vi "GSP_Manager_SCLNServer_Handler.vi"(4 "error in (no error)":errorcluster, 6 "Actions":T1) -> (0 "error out":errorcluster, 2 "reference out (launch only)":refnum<vi>)   [LabVIEW 2015]
uses:
  TCS_Link/TCSLINK_handler_actions.ctl
panel:
  out "Config filename":path=path "examples.cfg"
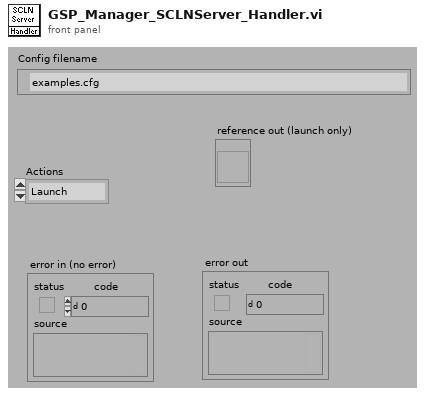
[diagram p1: front panel]
types:
  T1 = typedef "TCSLINK_handler_actions.ctl" = enum16{"Launch", "Shutdown"}
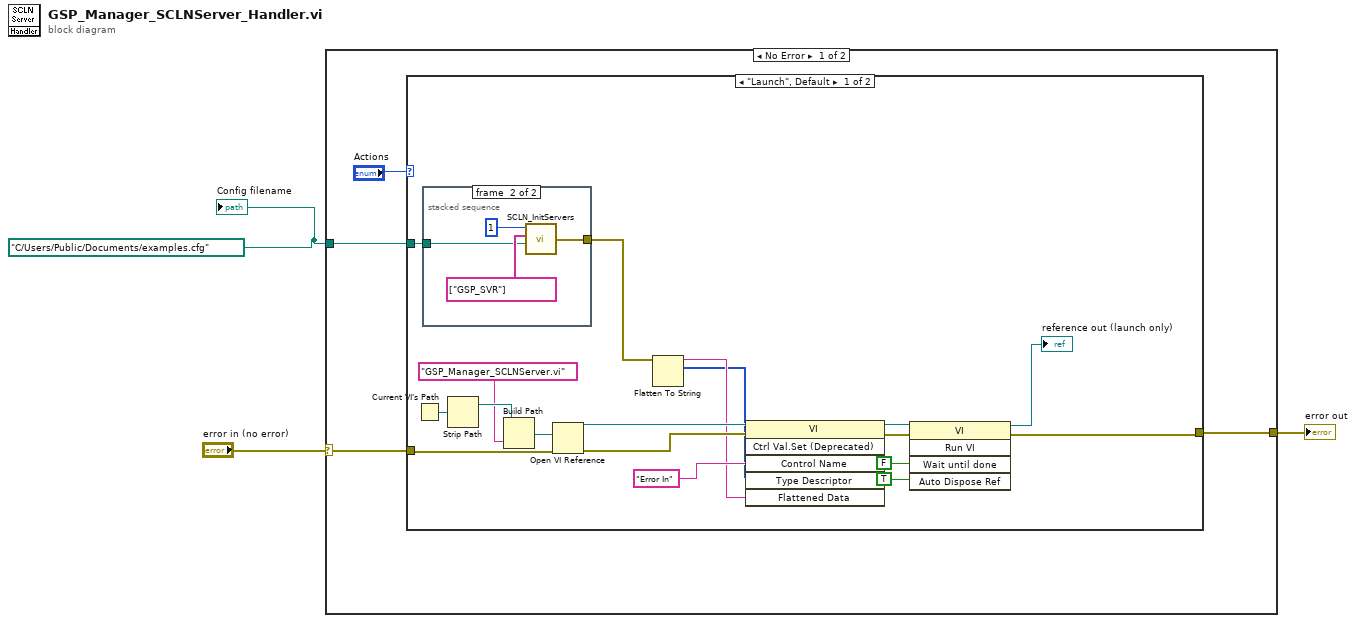
[diagram p0: block diagram]
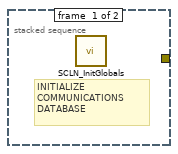
[diagram p2: hidden frame]
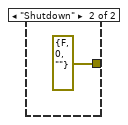
[diagram p3: hidden frame]
diagram:
  w1 = path "C:/Users/Public/Documents/examples.cfg"
  n1 = case shown="No Error" "error in (no error)" {
    selector: "error in (no error)" -> [w6 w31]
    tunnel: [w7 w31] -> w3
    tunnel: w1 -> [w4 _]
    frame No Error {
      n2 = case shown="\"Launch\", Default" "Actions" {
        tunnel: w6 -> [w25 _]
        tunnel: [w18 errorcluster {"status"=FALSE, "code"=0, "source"=""} ("error out")] -> w7
        tunnel: w4 -> [w8 _]
        frame "Launch", Default {
          n3 = Current VI's Path() -> (path=w22:path)
          n4 = stacked-sequence {
            tunnel: [_ w28] -> w9
            tunnel: w8 -> [_ w26]
            frame #0 {
              # "INITIALIZE\nCOMMUNICATIONS\nDATABASE"
              n5 = call "SCLN_InitGlobals.vi"() -> ()  [unwired: 1 in]
            }
            frame #1 {
              n6 = call "SCLN_InitServers.vi"("Config File Name"=w26, "Server Names"=string[] ["GSP_SVR"], "Num of Servers"=1) -> ("error out"=w28:errorcluster)  [unwired: 1 in]
            }
          }
          n7 = Strip Path(path=w22) -> (stripped path=w20:path)  [unwired: 1 out]
          n8 = Build Path(base path=w20, name or relative path="GSP_Manager_SCLNServer.vi" ("vi path")) -> (appended path=w21:path)
          n9 = Open VI Reference(vi path=w21, error in (no error)=w25) -> (vi reference=w14:refnum<vi>, error out=w13:errorcluster)  [unwired: 4 in]
          n10 = Flatten To String(anything=w9) -> (data string=w11:string, type string=w10:i16[])  [unwired: 3 in, 1 out]
          n11 = invoke class="VI" method="Ctrl Val.Set (Deprecated)"(reference=w14, error in=w13, "Control Name"="Error In", "Type Descriptor"=w10, "Flattened Data"=w11) -> (reference out=w16:refnum<vi>, error out=w15:errorcluster)  [unwired: 1 in, 4 out]
          n12 = invoke class="VI" method="Run VI"(reference=w16, error in=w15, "Wait until done"=FALSE, "Auto Dispose Ref"=TRUE) -> (reference out=→"reference out (launch only)":refnum<vi>, error out=w18:errorcluster)  [unwired: 1 in, 3 out]
        }
        frame "Shutdown" {
        }
      }
    }
    frame Error {
    }
  }
  "error out" <- w3
  "Config filename" <- w1
